vi "TailInsertionBenchmark_NativeArrayWithBoxing.vi"() -> ()   [LabVIEW 2013]
uses:
  source/LapDog.Collections.Common/String/String.lvclass
panel:
  out "Array":refnum<class "String.lvclass">[](array[class])
  in  "Number of Elements":i32
  out "Native Array":u32
  # "Tail Insertion - Native Array Boxing"
  # "100,000 to 500,000 elements is sufficient to see the difference in time for each of the implementations."
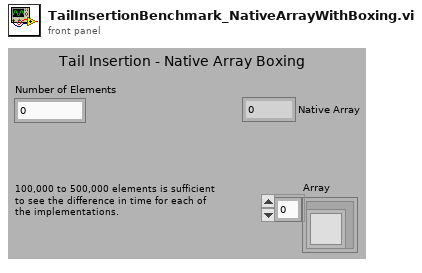
[diagram p1: front panel]
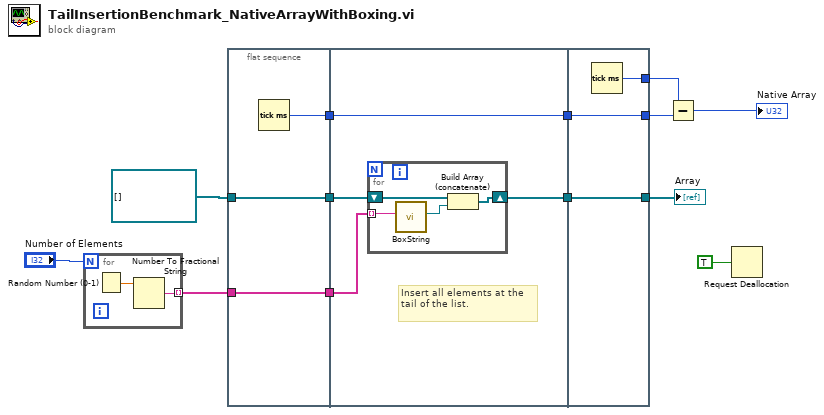
[diagram p0: block diagram]
diagram:
  n1 = for {
    N: "Number of Elements" -> [_]
    tunnel: [w14] -> w12 mode=indexing
    n2 = Random Number (0-1)() -> (number: 0 to 1=w15:dbl)
    n3 = Number To Fractional String(number=w15) -> (F-format string=w14:string)  [unwired: 3 in]
  }
  n4 = flat-sequence {
    tunnel: w12 -> [w18]
    tunnel: [w18] -> w11
    tunnel: [w17] -> w10
    tunnel: [w16] -> w9
    tunnel: refnum<class "String.lvclass">[] [] -> [w16]
    tunnel: w11 -> [w22]
    tunnel: w10 -> [w19]
    tunnel: w9 -> [w21]
    tunnel: [w20] -> w8
    tunnel: [w19] -> w7
    tunnel: [w29] -> w1
    tunnel: w8 -> [w29]
    tunnel: w7 -> [w27]
    tunnel: [w28] -> w6
    tunnel: [w27] -> w5
    frame #0 {
      n5 = Tick Count (ms)() -> (millisecond timer value=w17:u32)
    }
    frame #1 {
      # "Insert all elements at the tail of the list."
      n6 = for {
        shift-right: [w25] -> w20
        shift-left: w21 -> [w26]
        tunnel: w22 -> [w24] mode=indexing
        n7 = call "BoxString.vi"("String"=w24) -> ("String out"=w23:refnum<class "String.lvclass">)  [unwired: 10 in]
        n8 = Build Array (concatenate)(w26, w23) -> (w25:refnum<class "String.lvclass">[])
      }
    }
    frame #2 {
      n9 = Tick Count (ms)() -> (millisecond timer value=w28:u32)
    }
  }
  n10 = Subtract(x=w6, y=w5) -> (x-y=→"Native Array":u32)
  n11 = Request Deallocation(TRUE ("flag")) -> ()
  "Array" <- w1
